vi "niDTS WLAN INSTR TX Results Parse FSEG.vi"(11 "String":string="1,6,1,-20.980346,-29770408.163265,-91.302336,2,-12.698554,-18520408.163265,-86.544446,3,-6.935739,-11020408.163265,-85.640594,4,-6.138819,10867346.938776,-85.092842,5,-14.872167,18979591.836735,-84.778995,6,-20.937754,29005102.040816,-90.426561,2,6,1,-20.763251,-29770408.163265,-91.168959,2,-12.648617,-18520408.163265,-86.243912,3,-6.727863,-11020408.163265,-85.497999,4,-3.865118,10867346.938776,-87.016073,5,-14.432668,18979591.836735,-84.868024,6,-20.657802,29005102.040816,-90.356041") -> (3 "SEM:FSEGemts":T1)   [LabVIEW 2015, in "niDTS WLAN.lvlib" / "niDTS WLAN INSTR TX.lvclass"]
uses:
  niDTS WLAN INSTR TX.lvclass
  niDTS WLAN INSTR TX INC SEM FSEGemts Results.ctl
  Tests/Tx Test/Includes/Results/niDTS Tx RES INC SEM FSEGemts.ctl
  niDTS WLAN.lvlib
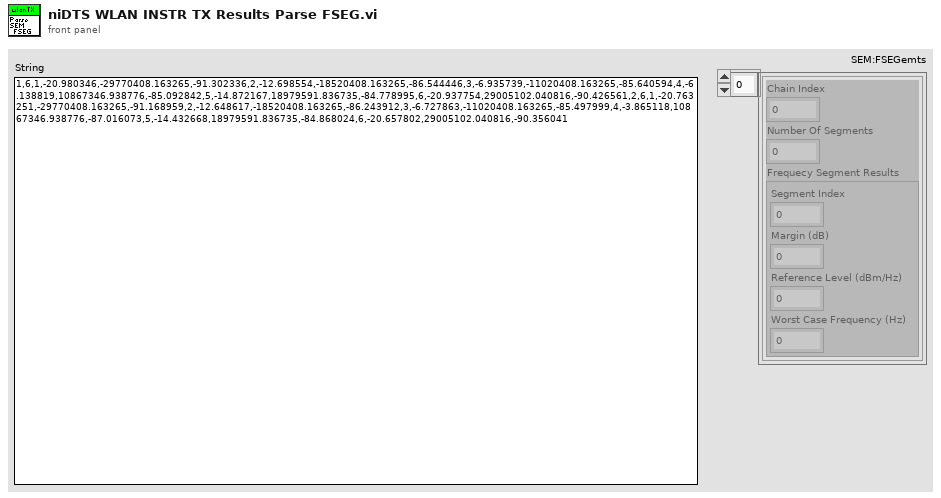
[diagram p1: front panel]
types:
  T1 = typedef "niDTS WLAN.lvlib/niDTS WLAN INSTR TX.lvclass/niDTS WLAN INSTR TX INC SEM FSEGemts Results.ctl" = T2[]
  T2 = typedef "niDTS WLAN.lvlib/niDTS Tx RES INC SEM FSEGemts.ctl" = cluster{"Chain Index":i32, "Number Of Segments":i32, "Frequecy Segment Results":cluster{"Segment Index":i32, "Margin (dB)":dbl, "Reference Level (dBm/Hz)":dbl, "Worst Case Frequency (Hz)":dbl}}
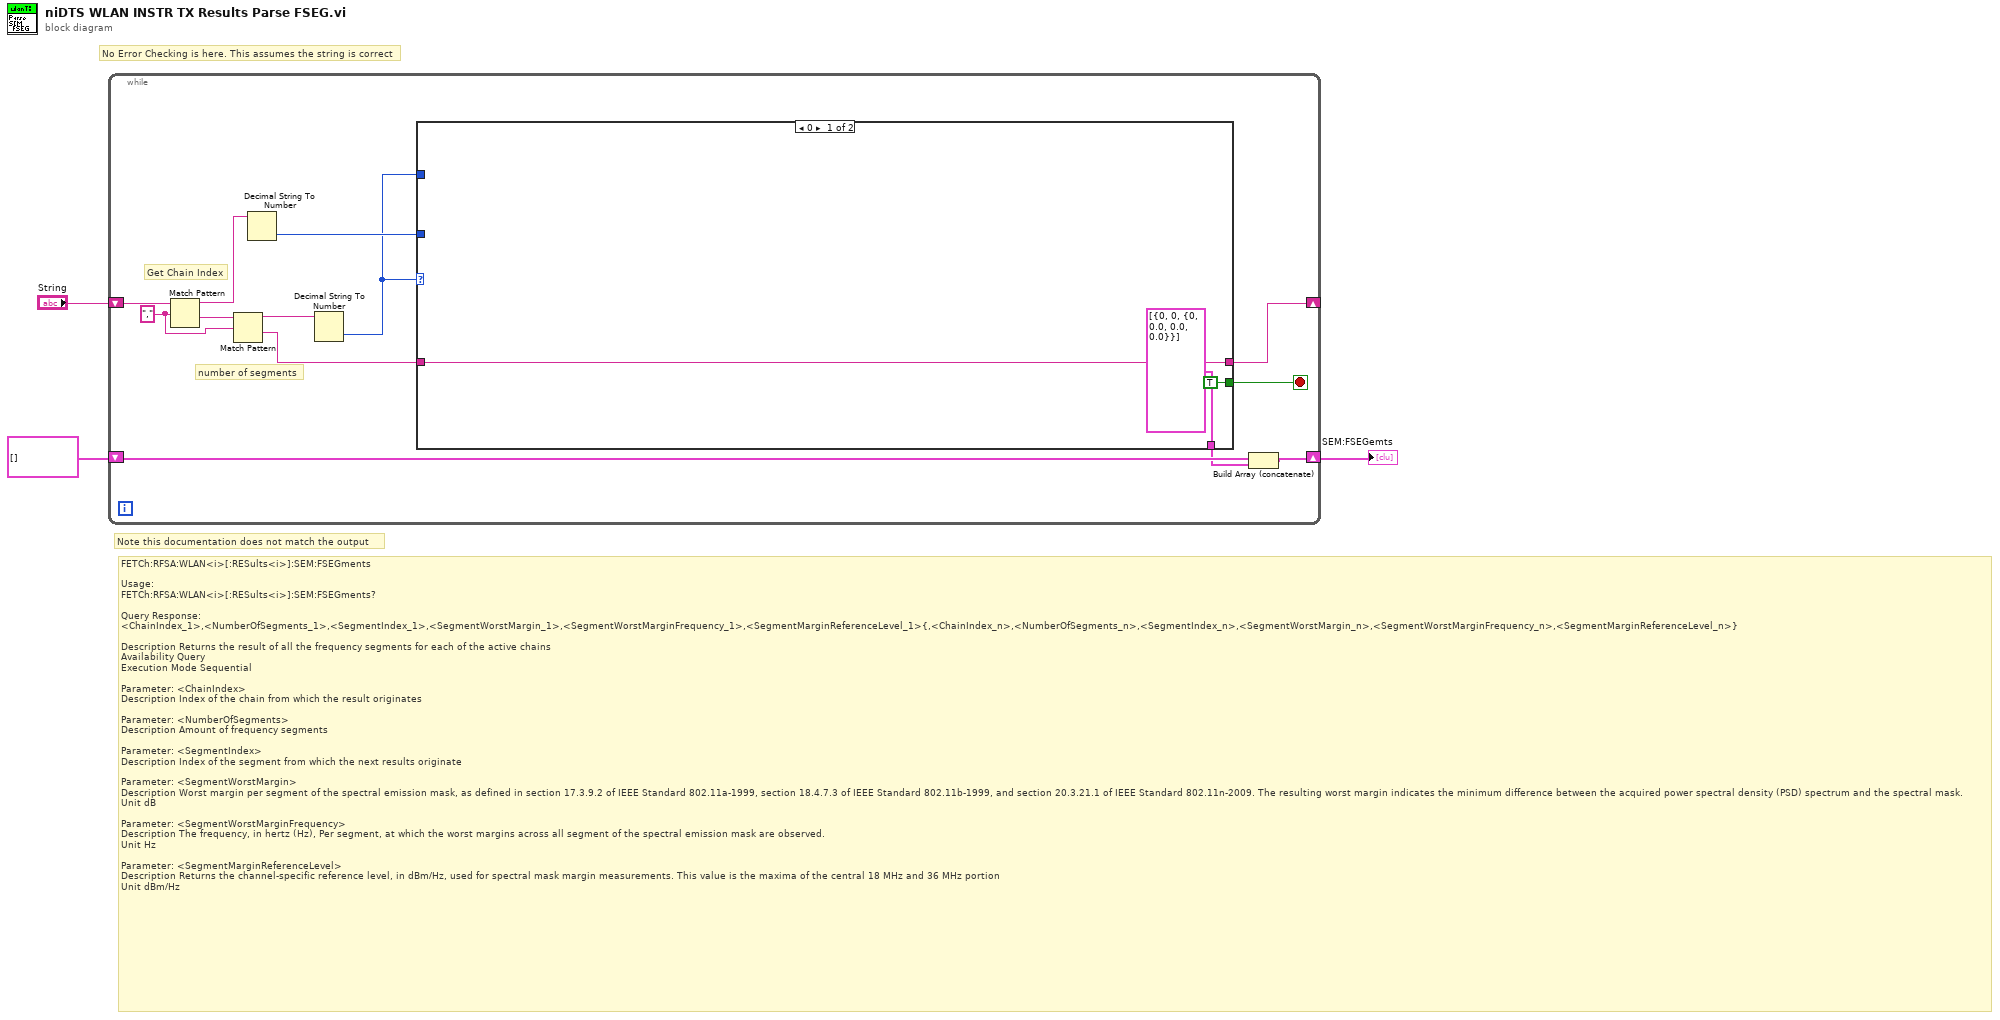
[diagram p0: block diagram]
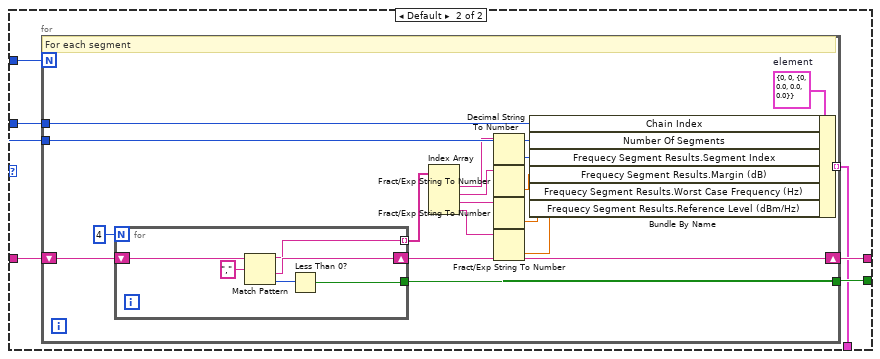
[diagram p2: hidden frame]
diagram:
  # "No Error Checking is here. This assumes the string is correct"
  # "Note this documentation does not match the output"
  # "FETCh:RFSA:WLAN<i>[:RESults<i>]:SEM:FSEGments\n\nUsage:\nFETCh:RFSA:WLAN<i>[:RESults<i>]:SEM:FSEGments? \n\nQuery Response:\n<ChainIndex_1>,<NumberOfSegments_1>,<SegmentIndex_1>,<SegmentWorstMargin_1>,<SegmentWorstMarginFrequency_1>,<SegmentMarginReferenceLevel_1>{,<ChainIndex_n>,<NumberOfSegments_n>,<SegmentIndex_n>,<SegmentWorstMargin_n>,<SegmentWorstMarginFrequency_n>,<SegmentMarginReferenceLevel_n>}\n\nDescription\tReturns the result of all the frequency segments for each of the active chains\nAvailability\tQuery\nExecution Mode\tSequential\n\nParameter: <ChainIndex>\nDescription\tIndex of the chain from which the result originates\n\nParameter: <NumberOfSegments>\nDescription\tAmount of frequency segments\n\nParameter: <SegmentIndex>\nDescription\tIndex of the segment from which the next results originate\n\nParameter: <SegmentWorstMargin>\nDescription\tWorst margin per segment of the spectral emission mask, as defined in section 17.3.9.2 of IEEE Standard 802.11a-1999, section 18.4.7.3 of IEEE Standard 802.11b-1999, and section 20.3.21.1 of IEEE Standard 802.11n-2009. The resulting worst margin indicates the minimum difference between the acquired power spectral density (PSD) spectrum and the spectral mask.\nUnit\tdB\n\nParameter: <SegmentWorstMarginFrequency>\nDescription\tThe frequency, in hertz (Hz), Per segment, at which the worst margins across all segment of the spectral emission mask are observed.\nUnit\tHz\n\nParameter: <SegmentMarginReferenceLevel>\nDescription\tReturns the channel-specific reference level, in dBm/Hz, used for spectral mask margin measurements. This value is the maxima of the central 18 MHz and 36 MHz portion\nUnit\tdBm/Hz"
  n1 = while {
    shift-right: [w10] -> _
    shift-left: "String" -> [w16]
    shift-right: [w5] -> w1
    shift-left: T1 [] ("SEM:FSEGemts") -> [w7]
    stop <- w11 stop-if-true
    w14 = "," ("search string/char (-)")
    # "number of segments"
    # "Get Chain Index"
    n2 = Match Pattern(string=w16, regular expression=w14) -> (before substring=w9:string, after substring=w15:string)  [unwired: 1 in, 2 out]
    n3 = Match Pattern(string=w15, regular expression=w14) -> (before substring=w13:string, after substring=w12:string)  [unwired: 1 in, 2 out]
    n4 = Decimal String To Number(string=w9) -> (number=w8:i32)  [unwired: 2 in, 1 out]
    n5 = Decimal String To Number(string=w13) -> (number=w4:i32)  [unwired: 2 in, 1 out]
    n6 = case shown="0" w4 {
      tunnel: w12 -> [w18 w25]
      tunnel: [TRUE w24] -> w11
      tunnel: [w18 w23] -> w10
      tunnel: w8 -> [_ w22]
      tunnel: w4 -> [_ w21]
      tunnel: [T2[] [{"Chain Index"=0, "Number Of Segments"=0, "Frequecy Segment Results"={"Segment Index"=0, "Margin (dB)"=0.0, "Reference Level (dBm/Hz)"=0.0, "Worst Case Frequency (Hz)"=0.0}}] w20] -> w6
      frame 0 {
      }
      frame Default {
        n7 = for {
          N: w21 -> [_]
          shift-right: [w40] -> w23
          shift-left: w25 -> [w42]
          tunnel: [w39] -> w24
          tunnel: w22 -> [w37]
          tunnel: w21 -> [w36]
          tunnel: [w26] -> w20 mode=indexing
          w38 = T2 {"Chain Index"=0, "Number Of Segments"=0, "Frequecy Segment Results"={"Segment Index"=0, "Margin (dB)"=0.0, "Reference Level (dBm/Hz)"=0.0, "Worst Case Frequency (Hz)"=0.0}}  # element
          # "For each segment"
          n8 = for {
            N: 4 -> [_]
            shift-right: [w45] -> w40
            shift-left: w42 -> [w48]
            tunnel: [w44] -> w35 mode=indexing
            tunnel: [w43] -> w39
            n9 = Match Pattern(string=w48, regular expression=",") -> (before substring=w44:string, after substring=w45:string, offset past match=w46:i32)  [unwired: 1 in, 1 out]
            n10 = Less Than 0?(x=w46) -> (x < 0?=w43:bool)
          }
          n11 = Index Array(array=w35) -> (element #1=w34:string, element #2=w32:string, element #3=w31:string, element #4=w30:string)  [unwired: 4 in]
          n12 = Decimal String To Number(string=w34) -> (number=w33:i32)  [unwired: 2 in, 1 out]
          n13 = Fract/Exp String To Number(string=w32) -> (number=w29:dbl)  [unwired: 3 in, 1 out]
          n14 = Fract/Exp String To Number(string=w31) -> (number=w28:dbl)  [unwired: 3 in, 1 out]
          n15 = Fract/Exp String To Number(string=w30) -> (number=w27:dbl)  [unwired: 3 in, 1 out]
          n16 = Bundle By Name(cluster=w38, "Chain Index"=w37, "Number Of Segments"=w36, "Frequecy Segment Results.Segment Index"=w33, "Frequecy Segment Results.Margin (dB)"=w29, "Frequecy Segment Results.Worst Case Frequency (Hz)"=w28, "Frequecy Segment Results.Reference Level (dBm/Hz)"=w27) -> (w26:T2)
        }
      }
    }
    n17 = Build Array (concatenate)(w7, w6) -> (w5:T1)
  }
  "SEM:FSEGemts" <- w1
